vi "RobotDLLHoming (SubVI).vi"(4 "Homing XYZ Stage":bool, 5 "Homing Tool":bool, 6 "Homing Arm":bool, 7 "ArmID":i32) -> (0 "Homing XYZ Stage Done":bool, 1 "Homing Tool Done":bool, 2 "Homing Arm Done":bool)   [LabVIEW 2016]
uses:
  EyeRobotDLL.dll
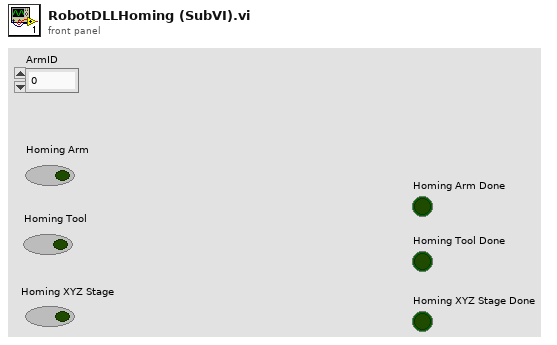
[diagram p1: front panel]
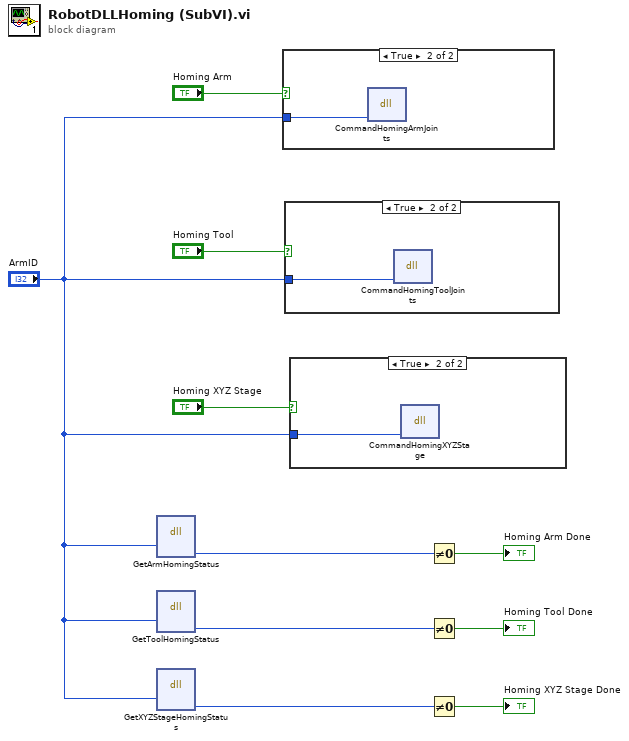
[diagram p0: block diagram]
diagram:
  n1 = dll-call lib="D:/IRISSoft LV2016 beta/Host Demo/Functions/EyeRobotDLL.dll" fn="GetArmHomingStatus"("id"="ArmID") -> ("status"=w5:u8)  [unwired: 6 in, 2 out]
  n2 = dll-call lib="D:/IRISSoft LV2016 beta/Host Demo/Functions/EyeRobotDLL.dll" fn="GetToolHomingStatus"("id"="ArmID") -> ("status"=w4:u8)  [unwired: 6 in, 2 out]
  n3 = dll-call lib="D:/IRISSoft LV2016 beta/Host Demo/Functions/EyeRobotDLL.dll" fn="GetXYZStageHomingStatus"("id"="ArmID") -> ("status"=w3:u8)  [unwired: 6 in, 2 out]
  n4 = case shown="True" "Homing Arm" {
    tunnel: "ArmID" -> [_ w11]
    frame False {
    }
    frame True {
      n5 = dll-call lib="D:/IRISSoft LV2016 beta/Host Demo/Functions/EyeRobotDLL.dll" fn="CommandHomingArmJoints"("id"=w11) -> ()  [unwired: 5 in, 2 out]
    }
  }
  n6 = case shown="True" "Homing Tool" {
    tunnel: "ArmID" -> [_ w12]
    frame False {
    }
    frame True {
      n7 = dll-call lib="D:/IRISSoft LV2016 beta/Host Demo/Functions/EyeRobotDLL.dll" fn="CommandHomingToolJoints"("id"=w12) -> ()  [unwired: 5 in, 2 out]
    }
  }
  n8 = case shown="True" "Homing XYZ Stage" {
    tunnel: "ArmID" -> [_ w13]
    frame False {
    }
    frame True {
      n9 = dll-call lib="D:/IRISSoft LV2016 beta/Host Demo/Functions/EyeRobotDLL.dll" fn="CommandHomingXYZStage"("id"=w13) -> ()  [unwired: 5 in, 2 out]
    }
  }
  n10 = Not Equal To 0?(x=w5) -> (x != 0?=→"Homing Arm Done":bool)
  n11 = Not Equal To 0?(x=w4) -> (x != 0?=→"Homing Tool Done":bool)
  n12 = Not Equal To 0?(x=w3) -> (x != 0?=→"Homing XYZ Stage Done":bool)
